vi "calc ROI.vi"(11 "Image":T1(plugin-control)) -> (3 "only ROI Cluster":T2)   [LabVIEW 2011]
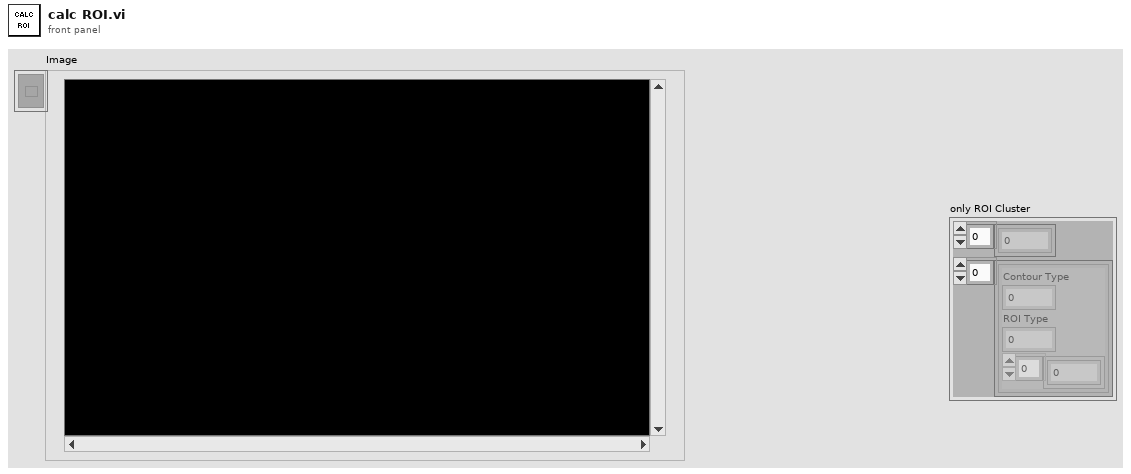
[diagram p1: front panel]
types:
  T1 = typedef "IMAQ Image.ctl" = refnum<image>
  T2 = cluster{i32[], cluster{"Contour Type":u32, "ROI Type":u32, i32[]}[]}
  T3 = cluster{"Contour Type":u32, "ROI Type":u32, i32[]}
  T4 = cluster{"Contour Type":u32, "ROI Type":u32, i32[]}[]
  T5 = cluster{"Global Rectangle":i32[], "Contours":cluster{"Contour Type":u32, "ROI Type":u32, "Points":i32[]}[]}
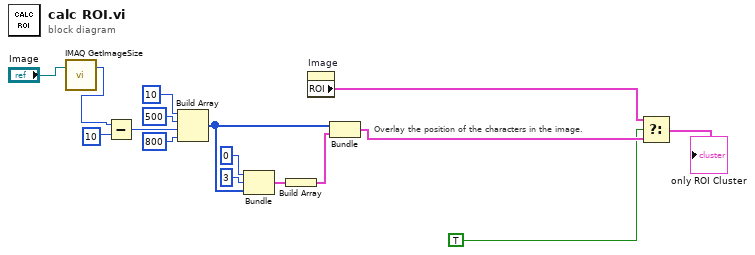
[diagram p0: block diagram]
diagram:
  # "Overlay the position of the characters in the image."
  n1 = call "IMAQ GetImageSize"("Image"="Image") -> ("Y Resolution"=w6:i32)  [unwired: 3 in, 2 out]
  n2 = Subtract(x=w6, y=10) -> (x-y=w15:i32)
  n3 = Build Array(10 ("element"), 500 ("element"), w15, 800 ("element")) -> (w12:i32[])
  n4 = Bundle("Contour Type"=u32 0, "ROI Type"=u32 3, w12) -> (w10:T3)  [unwired: 1 in]
  n5 = Build Array(w10) -> (w11:T4)
  n6 = property on="Image" class="ImageControl"() -> ("ROI"=w3:T5)  [unwired: 2 in, 2 out]
  n7 = Bundle(w12, w11) -> (w2:T2)  [unwired: 1 in]
  n8 = Select(t=w3, s=TRUE, f=w2) -> (s? t:f=→"only ROI Cluster":T5)
